vi "Play Video From File.vi"() -> ()   [LabVIEW 2018]
doc: "Play Video From File: This example is an example of calling a file video, which can find and play the video from a local file for the next visual processing step."
uses:
  vi.lib/VIRobotics/opencv_yiku/ctls/ColorConversionCodes.ctl
  vi.lib/VIRobotics/opencv_yiku/Mat/Mat_8U/Mat_8U.lvclass
  D:/Program Files/company/National Instruments/LabVIEW 2018/vi.lib/addons/VIRobotics/opencv_yiku/Mat/Mat/Mat.lvclass
  vi.lib/VIRobotics/opencv_yiku/Mat/Create_Mat_8U.vi
  vi.lib/VIRobotics/opencv_yiku/Cap/Cap.lvclass
  vi.lib/VIRobotics/opencv_yiku/opencv_yiku.lvlib
panel:
  in  "video file":string="test.mp4"
  out "picture":picture
  in  "stop":bool
  # "Overview: Demonstrates how to play a video from the file\nRequirements: Windows.\nInstructions: \n1. Run the VI"
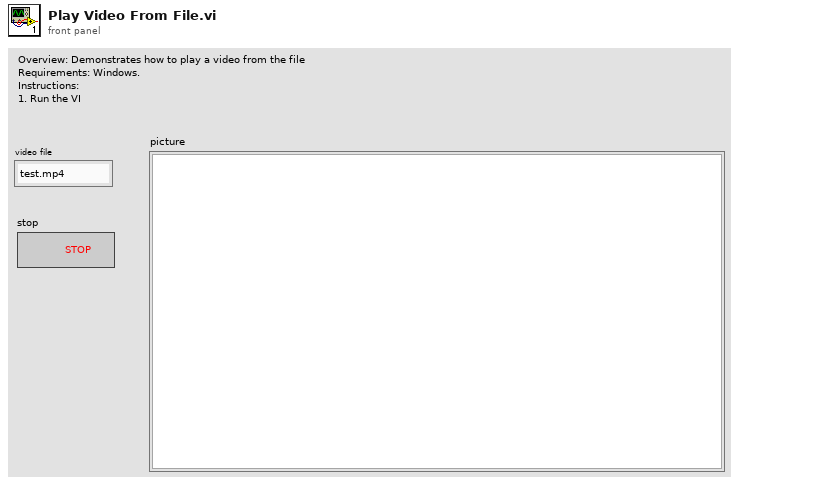
[diagram p1: front panel]
types:
  T1 = typedef "opencv_yiku.lvlib/ColorConversionCodes.ctl" = enum32{"COLOR_BGR2BGRA", "COLOR_BGRA2BGR", "COLOR_BGR2RGBA", "COLOR_RGBA2BGR", "COLOR_BGR2RGB", "COLOR_BGRA2RGBA", "COLOR_BGR2GRAY", "COLOR_RGB2GRAY", "COLOR_GRAY2BGR", "COLOR_GRAY2BGRA", "COLOR_BGRA2GRAY", "COLOR_RGBA2GRAY", "COLOR_BGR2BGR565", "COLOR_RGB2BGR565", "COLOR_BGR5652BGR", "COLOR_BGR5652RGB", "COLOR_BGRA2BGR565", "COLOR_RGBA2BGR565", "COLOR_BGR5652BGRA", "COLOR_BGR5652RGBA", "COLOR_GRAY2BGR565", "COLOR_BGR5652GRAY", "COLOR_BGR2BGR555", "COLOR_RGB2BGR555", "COLOR_BGR5552BGR", "COLOR_BGR5552RGB", "COLOR_BGRA2BGR555", "COLOR_RGBA2BGR555", "COLOR_BGR5552BGRA", "COLOR_BGR5552RGBA", "COLOR_GRAY2BGR555", "COLOR_BGR5552GRAY", "COLOR_BGR2XYZ", "COLOR_RGB2XYZ", "COLOR_XYZ2BGR", "COLOR_XYZ2RGB", "COLOR_BGR2YCrCb", "COLOR_RGB2YCrCb", "COLOR_YCrCb2BGR", "COLOR_YCrCb2RGB", "COLOR_BGR2HSV", "COLOR_RGB2HSV", "42", "43", "COLOR_BGR2Lab", "COLOR_RGB2Lab"}
  T2 = typedef "LVBoundsTypeDef.ctl" = cluster{"Width":u32, "Height":u32}
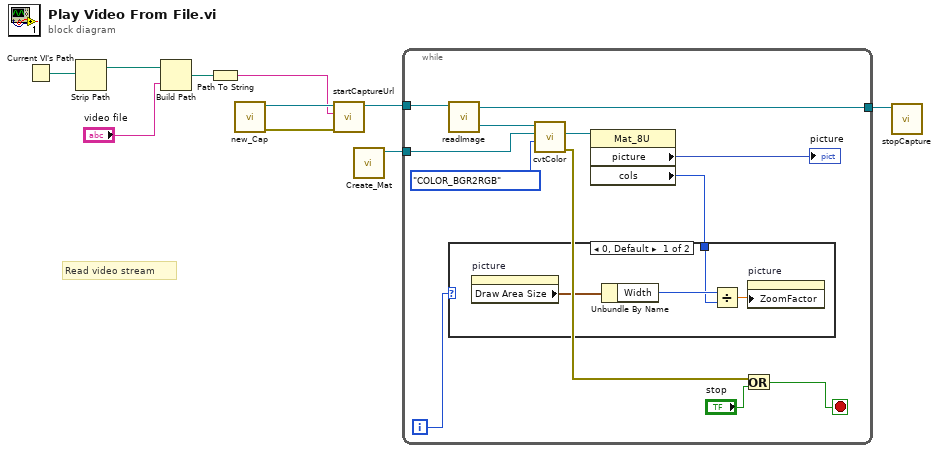
[diagram p0: block diagram]
diagram:
  # "Read video stream"
  n1 = Current VI's Path() -> (path=w4:path)
  n2 = Strip Path(path=w4) -> (stripped path=w5:path)  [unwired: 1 out]
  n3 = Build Path(base path=w5, name or relative path="video file") -> (appended path=w3:path)
  n4 = Path To String(path=w3) -> (string=w1:string)
  n5 = call "new_Cap.vi"() -> ("error out"=w7:errorcluster, "Cap out"=w8:refnum<class "Cap.lvclass">)  [unwired: 10 in]
  n6 = call-dynamic "startCaptureUrl.vi"("error in (no error)"=w7, "url"=w1, "Cap in"=w8) -> ("Cap out"=w6:refnum<class "Cap.lvclass">)  [unwired: 7 in, 1 out]
  n7 = call-poly "Create_Mat.vi"() -> ("Mat_8U_out"=w9:refnum<class "Mat_8U.lvclass">)  [unwired: 10 in, 1 out]
  n8 = while {
    tunnel: w6 -> [w22]
    tunnel: [w21] -> w10
    tunnel: w9 -> [w19]
    i -> [w12]
    stop <- w13 stop-if-true
    n9 = call "readImage.vi"("Cap in"=w22) -> ("Mat out"=w20:refnum<class "Mat_8U.lvclass">, "Cap out"=w21:refnum<class "Cap.lvclass">)  [unwired: 8 in, 1 out]
    n10 = call "cvtColor.vi"("dstCn"=ColorConversionCodes."COLOR_BGR2RGB", "dst"=w19, "src"=w20) -> ("error out"=w14:errorcluster, "dst out"=w18:refnum<class "Mat_8U.lvclass">)  [unwired: 6 in, 1 out]
    n11 = property class="Mat_8U"(reference=w18) -> ("picture"=→"picture":picture, "cols"=w11:i32)  [unwired: 1 in, 2 out]
    n12 = case shown="0, Default" w12 {
      tunnel: w11 -> [w25 _]
      frame 0, Default {
        n13 = property on="picture" class="Pict"() -> ("Draw Area Size"=w24:T2)  [unwired: 2 in, 2 out]
        n14 = Unbundle By Name(w24) -> ("Width"=w26:u32)
        n15 = Divide(x=w26, y=w25) -> (x/y=w23:dbl)
        n16 = property on="picture" class="Pict"("ZoomFactor"=w23) -> ()  [unwired: 2 in, 2 out]
      }
      frame 1 {
      }
    }
    n17 = Or(x=w14, y="stop") -> (x .or. y?=w13:bool)
  }
  n18 = call "stopCapture.vi"("Cap in"=w10) -> ()  [unwired: 10 in, 1 out]
